vi "Pomiar_glowny.vi"() -> ()   [LabVIEW 2012]
panel:
  in  "stop":bool
  in  "Temp1":path
  in  "Temp2":path=path "D:/temperature2.txt"
  out "Temp 2 °C]":dbl format="%#_4g"
  out "Temp2 Chart":dbl(graph) caption="Temperature Chart"
  out "error out 2":errorcluster
  out "error out":errorcluster
  out "id":bool
  out "crc":bool
  out "Voltage [V]":dbl format="%#_2g"
  out "Potentiometer":dbl(knob) scale=0.0..3.0
  out "Temp1 Chart":dbl(graph) caption="Temperature Chart"
  out "Temp1 °C]":dbl format="%#_4g"
  out "Temp1":dbl(slide) scale=-40.0..120.0
  in  "Serial Port":refnum<visa-resource-name>="COM6"
  in  "stop":bool
  out "Received":string
  in  "?":bool
  # "POMIAR WARTOŒCI ANALOGOWYCH"
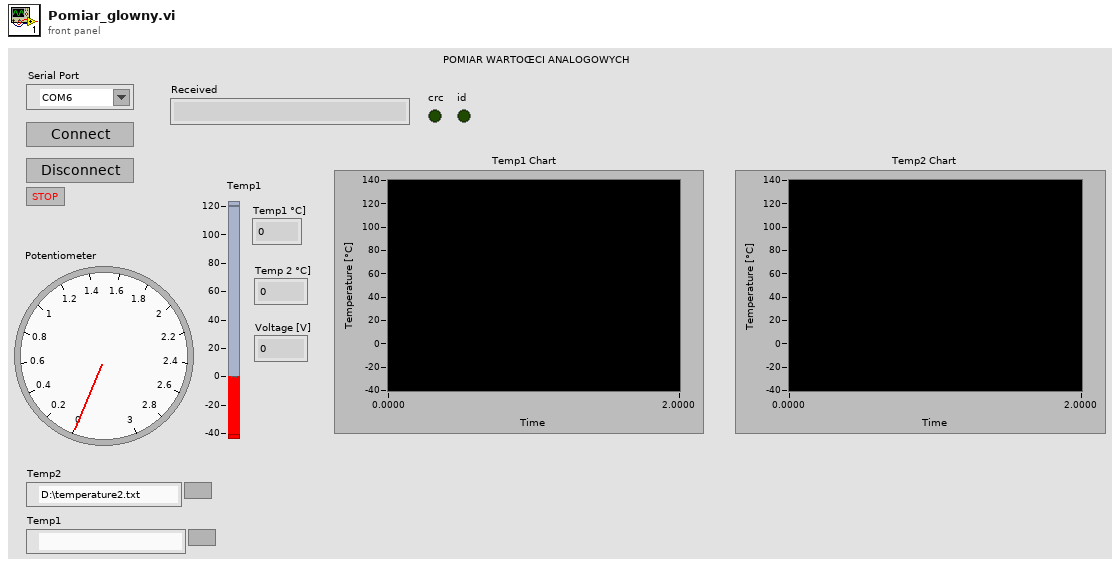
[diagram p1: front panel]
types:
  T1 = enum16{"open", "replace", "create", "open or create", "replace or create", "replace or create with confirmation"}
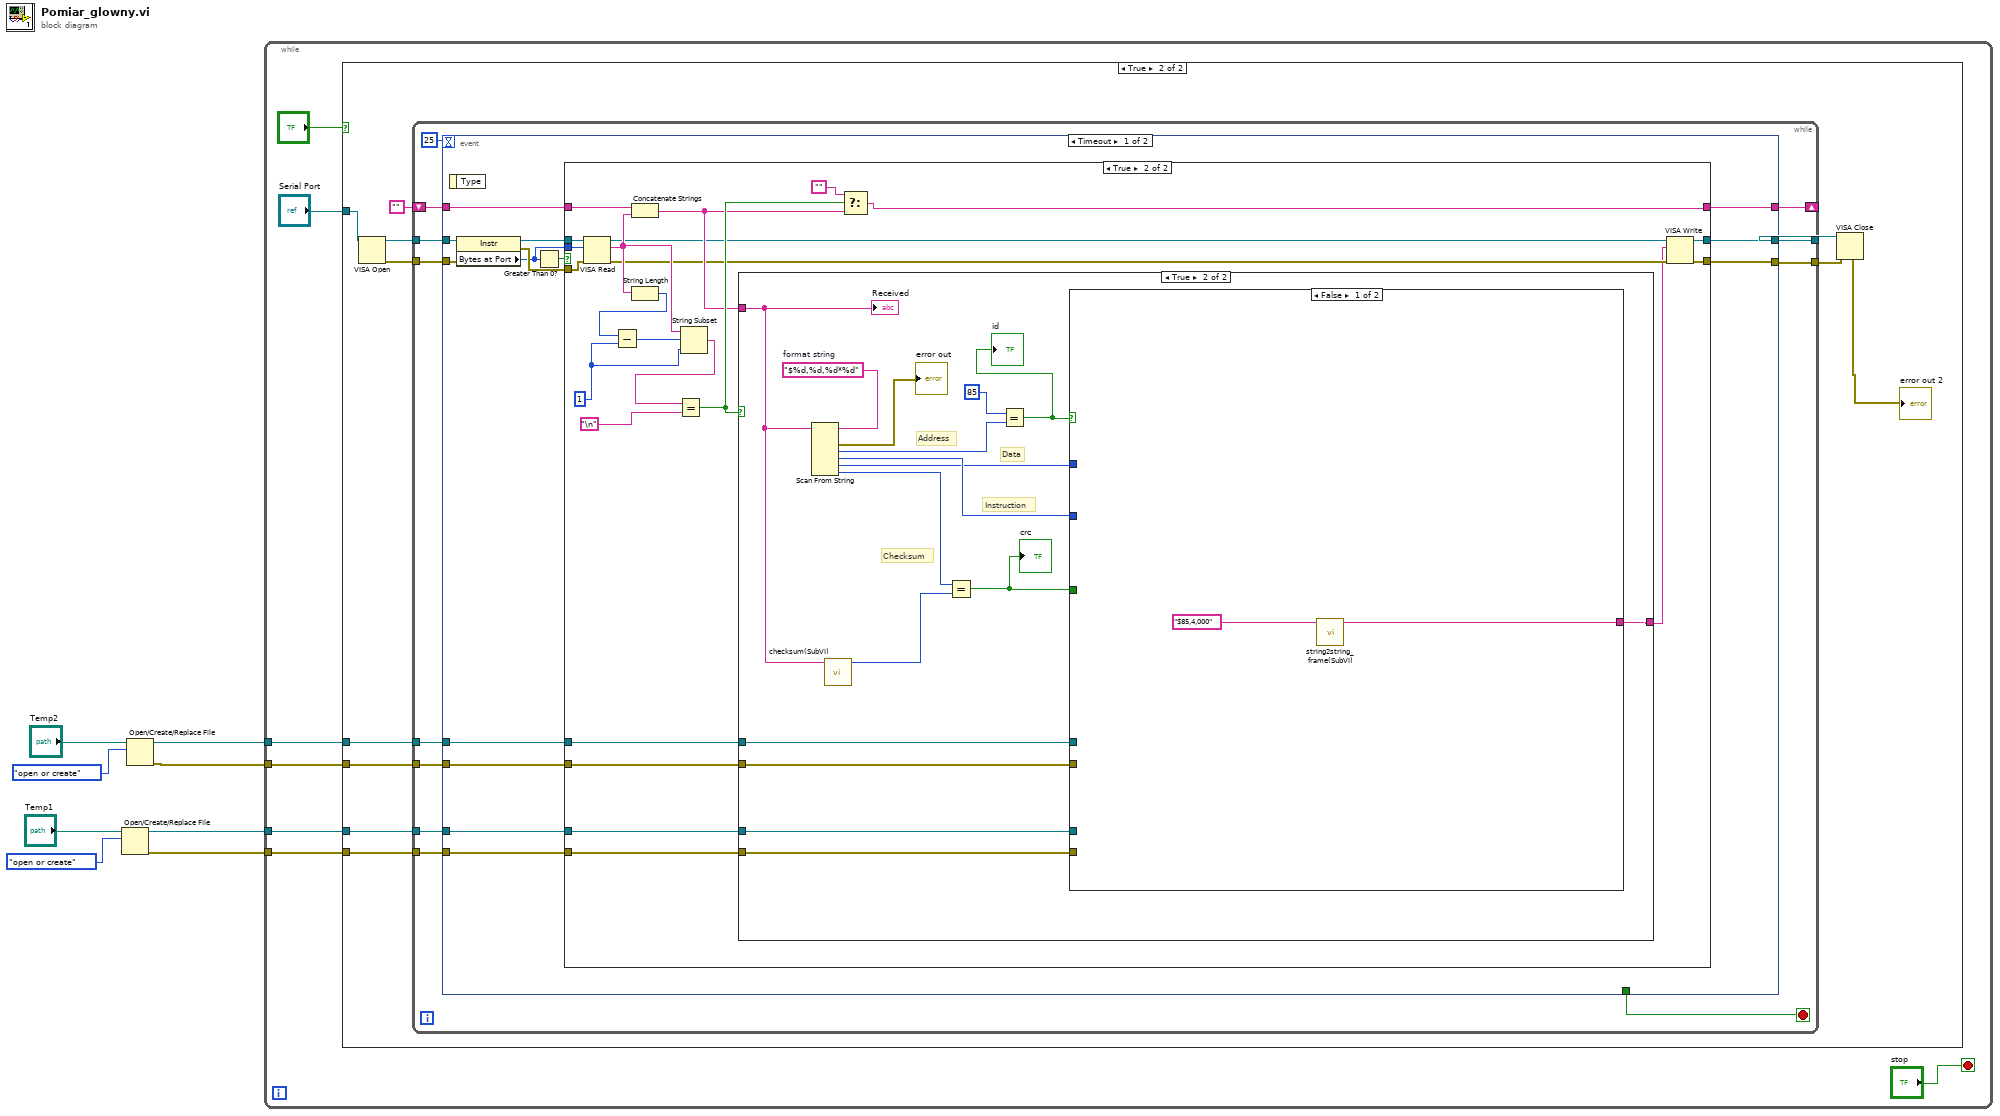
[diagram p0: block diagram]
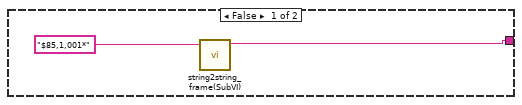
[diagram p4: hidden frame]
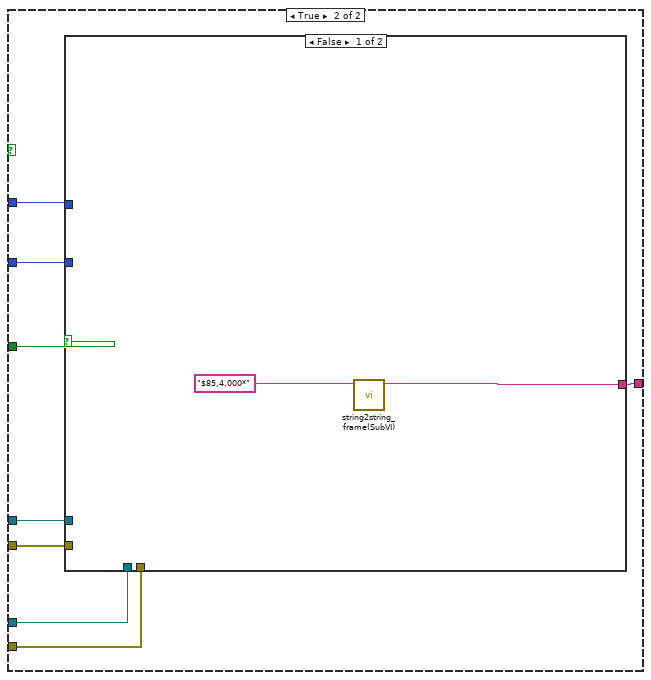
[diagram p5: hidden frame]
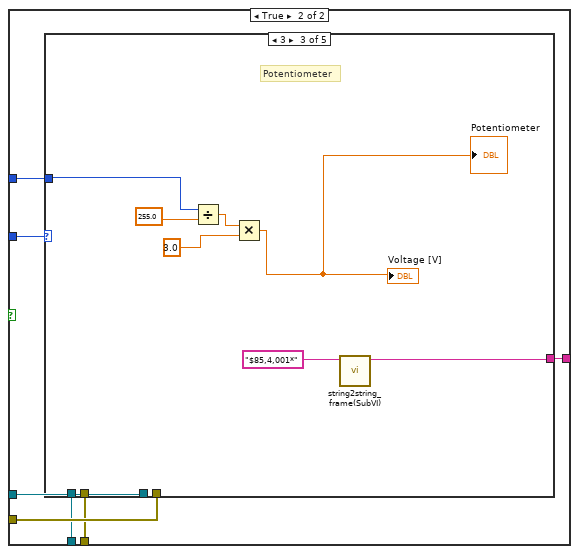
[diagram p6: hidden frame]
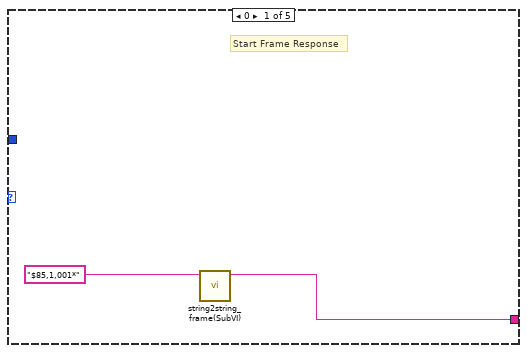
[diagram p7: hidden frame]
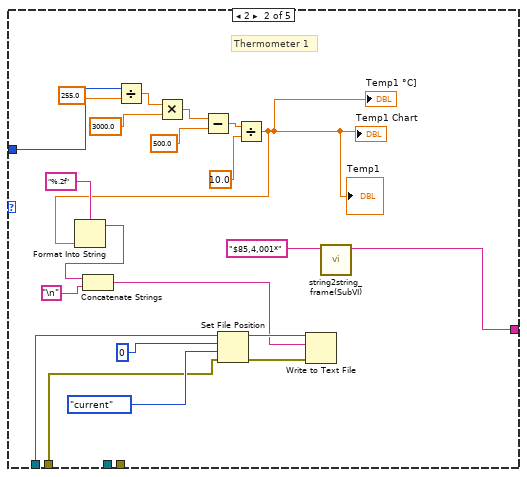
[diagram p8: hidden frame]
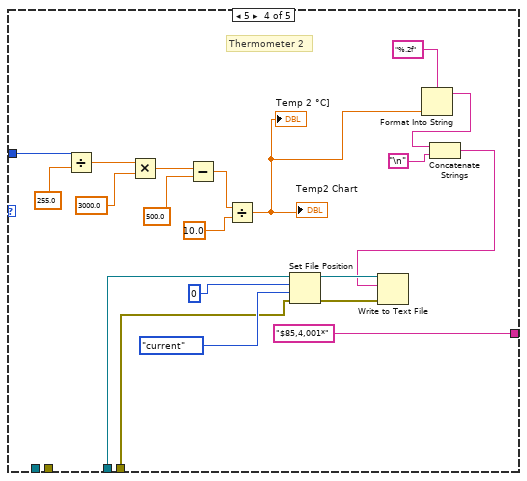
[diagram p9: hidden frame]
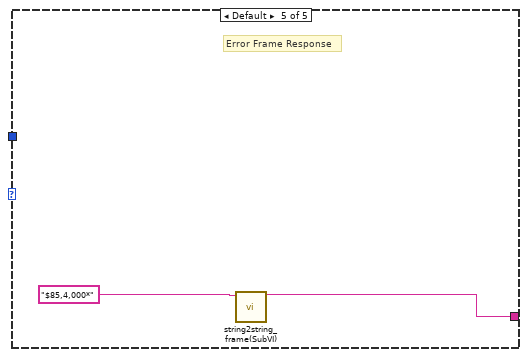
[diagram p10: hidden frame]
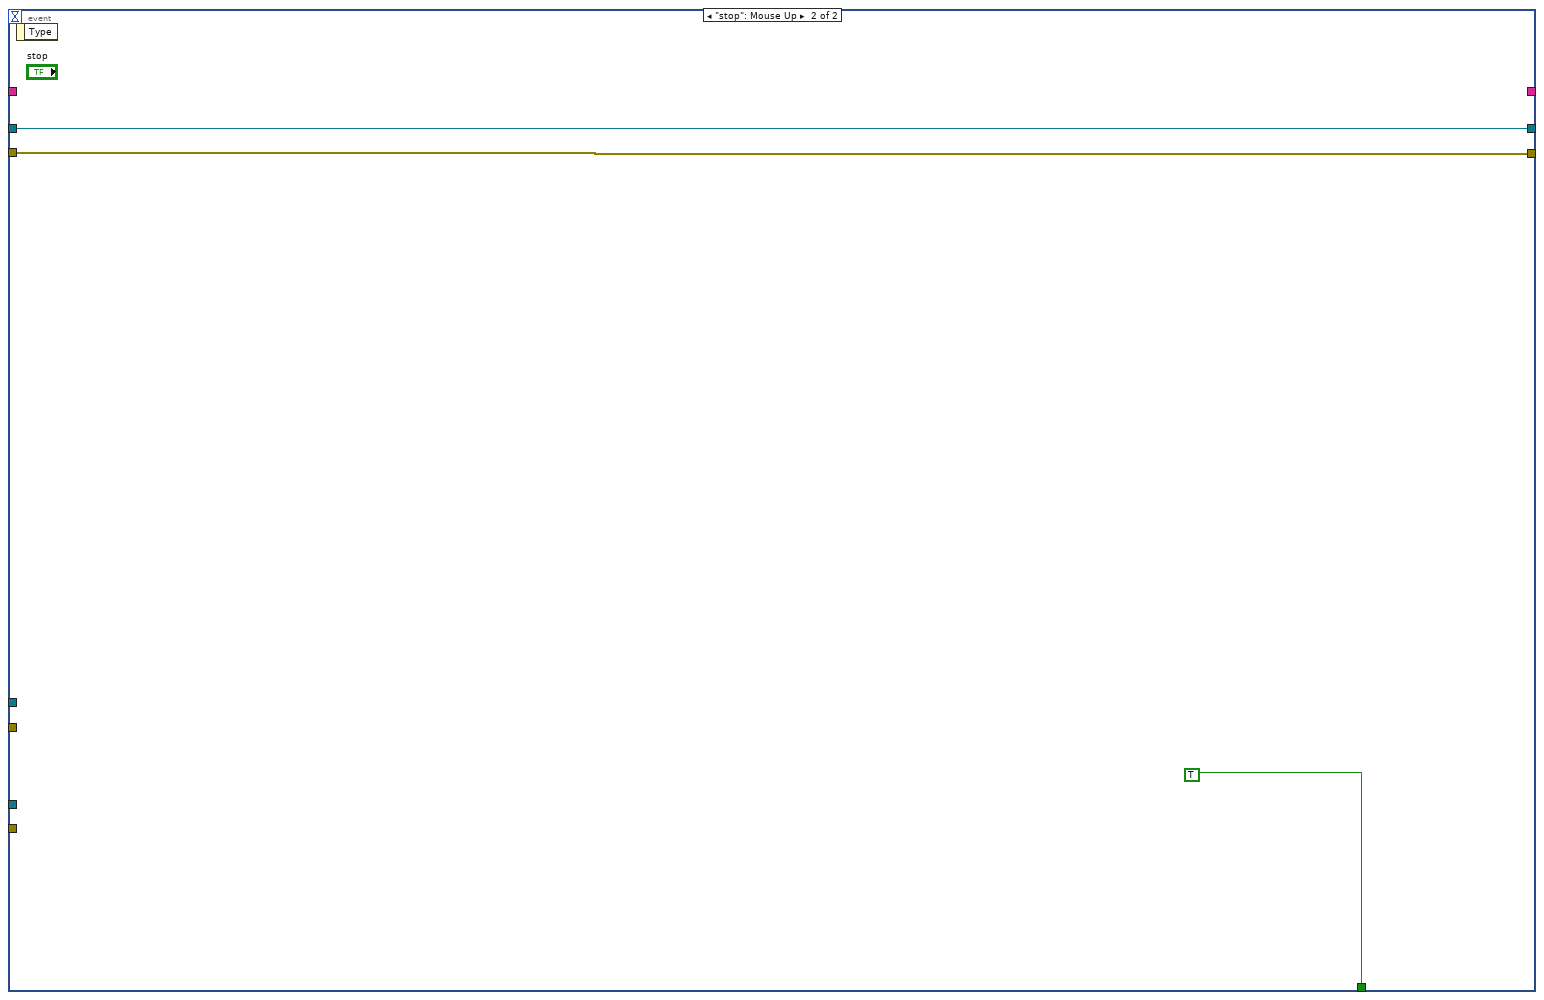
[diagram p11: hidden frame]
diagram:
  n1 = Open/Create/Replace File(file path (use dialog)="Temp1", operation (0:open)=T1."open or create") -> (refnum out=w2:refnum<file>, error out=w1:errorcluster)  [unwired: 4 in, 1 out]
  n2 = Open/Create/Replace File(file path (use dialog)="Temp2", operation (0:open)=T1."open or create") -> (refnum out=w6:refnum<file>, error out=w5:errorcluster)  [unwired: 4 in, 1 out]
  n3 = while {
    tunnel: w6 -> [w13]
    tunnel: w5 -> [w12]
    tunnel: w2 -> [w11]
    tunnel: w1 -> [w10]
    stop <- "stop" stop-if-true
    n4 = case shown="True" "?" {
      tunnel: "Serial Port" -> [_ w21]
      tunnel: w13 -> [_ w19]
      tunnel: w12 -> [_ w18]
      tunnel: w11 -> [_ w17]
      tunnel: w10 -> [_ w16]
      frame False {
      }
      frame True {
        n5 = VISA Open(VISA resource name=w21) -> (VISA resource name=w24:refnum<visa-resource-name>, error out=w23:errorcluster)  [unwired: 4 in]
        n6 = while {
          tunnel: w24 -> [w38]
          tunnel: [w37] -> w26
          tunnel: w23 -> [w35]
          tunnel: [w34] -> w25
          shift-right: [w32] -> _
          shift-left: "" -> [w33]
          tunnel: w19 -> [w30]
          tunnel: w18 -> [w29]
          tunnel: w17 -> [w28]
          tunnel: w16 -> [w27]
          stop <- w31 stop-if-true
          n7 = event shown="[0] Timeout" {
            selector: _ -> [_ _]
            dyn-events: _ -> [_ _]
            timeout: 25 ("millisecond multiple") -> [_ _]
            tunnel: w38 -> [w51 w170]
            tunnel: [w44 w170] -> w37
            tunnel: [_ TRUE] -> w31
            tunnel: w35 -> [w47 w168]
            tunnel: [w43 w168] -> w34
            tunnel: w33 -> [w46 _]
            tunnel: [w45 _] -> w32
            tunnel: w30 -> [w42 _]
            tunnel: w29 -> [w41 _]
            tunnel: w28 -> [w40 _]
            tunnel: w27 -> [w39 _]
            event Timeout {
              n8 = event-data() -> ()  [unwired: 1 in, 1 out]
              n9 = property class="Instr"(reference=w51, error in=w47) -> (reference out=w50:refnum<visa-resource-name>, error out=w52:errorcluster, "Bytes at Port"=w48:u32)
              n10 = Greater Than 0?(x=w48) -> (x > 0?=w49:bool)
              n11 = case shown="True" w49 {
                tunnel: w50 -> [w55 w78]
                tunnel: w48 -> [_ w77]
                tunnel: [w55 w64] -> w44
                tunnel: w52 -> [w53 w73]
                tunnel: w46 -> [w54 w72]
                tunnel: [w54 w70] -> w45
                tunnel: [w53 w63] -> w43
                tunnel: w42 -> [_ w59]
                tunnel: w41 -> [_ w58]
                tunnel: w40 -> [_ w57]
                tunnel: w39 -> [_ w56]
                frame False {
                }
                frame True {
                  w75 = 1 ("length (rest)")
                  n12 = VISA Read(VISA resource name=w78, byte count=w77, error in (no error)=w73) -> (VISA resource name out=w62:refnum<visa-resource-name>, read buffer=w74:string, error out=w61:errorcluster)  [unwired: 1 out]
                  n13 = Concatenate Strings(w72, w74) -> (w68:string)
                  n14 = String Length(string=w74) -> (length=w67:i32)
                  n15 = Subtract(x=w67, y=w75) -> (x-y=w76:i32)
                  n16 = String Subset(string=w74, offset (0)=w76, length (rest)=w75) -> (substring=w66:string)
                  n17 = Equal?(x=w66, y="\n") -> (x = y?=w69:bool)
                  n18 = case shown="True" w69 {
                    tunnel: w68 -> [_ w92]
                    tunnel: [w79 w88] -> w60
                    tunnel: w59 -> [_ w84]
                    tunnel: w58 -> [_ w83]
                    tunnel: w57 -> [_ w82]
                    tunnel: w56 -> [_ w81]
                    frame False {
                      n19 = call "string2string_frame(SubVI).vi"("String in"="$85,1,001*") -> ("String out"=w79:string)  [unwired: 10 in]
                    }
                    frame True {
                      w96 = "$%d,%d,%d*%d"  # format string
                      # "Checksum"
                      # "Instruction"
                      # "Data"
                      # "Address"
                      n20 = Scan From String(format string=w96, input string=w92) -> (error out=→"error out":errorcluster, output 1=w94:i32, output 2=w93:i32, output 3=w87:i32, output 4=w91:i32)  [unwired: 6 in, 2 out]
                      n21 = call "checksum(SubVI).vi"("String"=w92) -> ("Numeric"=w89:u8)  [unwired: 10 in]
                      n22 = Equal?(x=w91, y=w89) -> (x = y?=w86:bool)
                      "crc" <- w86
                      n23 = Equal?(x=85, y=w94) -> (x = y?=w90:bool)
                      "id" <- w90
                      n24 = case shown="False" w90 {
                        tunnel: w93 -> [_ w105]
                        tunnel: w87 -> [_ w106]
                        tunnel: w86 -> [_ w103]
                        tunnel: [w97 w104] -> w88
                        tunnel: w84 -> [_ w102]
                        tunnel: w83 -> [_ w101]
                        tunnel: w82 -> [_ w100]
                        tunnel: w81 -> [_ w99]
                        frame False {
                          n25 = call "string2string_frame(SubVI).vi"("String in"="$85,4,000") -> ("String out"=w97:string)  [unwired: 10 in]
                        }
                        frame True {
                          n26 = case shown="False" w103 {
                            tunnel: w106 -> [_ w115]
                            tunnel: w105 -> [_ w114]
                            tunnel: [w107 w113] -> w104
                            tunnel: w102 -> [_ w112]
                            tunnel: w101 -> [_ w111]
                            tunnel: w100 -> [_ w110]
                            tunnel: w99 -> [_ w109]
                            frame False {
                              n27 = call "string2string_frame(SubVI).vi"("String in"="$85,4,000*") -> ("String out"=w107:string)  [unwired: 10 in]
                            }
                            frame True {
                              n28 = case shown="3" w114 {
                                tunnel: w115 -> [_ w129 w140 w158 _]
                                tunnel: [w116 w131 w141 "$85,4,001*" w167] -> w113
                                tunnel: w112 -> [_ _ _ w148 _]
                                tunnel: w111 -> [_ _ _ w147 _]
                                tunnel: w110 -> [_ w124 _ _ _]
                                tunnel: w109 -> [_ w123 _ _ _]
                                frame 0 {
                                # "Start Frame Response"
                                n29 = call "string2string_frame(SubVI).vi"("String in"="$85,1,001*") -> ("String out"=w116:string)  [unwired: 10 in]
                                }
                                frame 2 {
                                # "Thermometer 1"
                                n30 = Divide(x=w129, y=255.0) -> (x/y=w137:dbl)
                                n31 = Multiply(x=w137, y=3000.0) -> (x*y=w135:dbl)
                                n32 = Subtract(x=w135, y=500.0) -> (x-y=w132:dbl)
                                n33 = Set File Position(offset (in bytes) (0)=u32 0 ("millisecond multiple"), refnum=w124, from (0:start)=enum16{"start", "end", "current"}."current", error in=w123) -> (refnum out=w126:refnum<file>, error out=w125:errorcluster)
                                n34 = Divide(x=w132, y=10.0) -> (x/y=w119:dbl)
                                "Temp1 Chart" <- w119
                                "Temp1 °C]" <- w119
                                "Temp1" <- w119
                                n35 = Format Into String(format string="%.2f", w119) -> (resulting string=w121:string)  [unwired: 2 in, 1 out]
                                n36 = Concatenate Strings(w121, "\n" ("Line Feed Constant")) -> (w118:string)
                                n37 = Write to Text File(file (use dialog)=w126, text=w118, error in=w125) -> ()  [unwired: 1 in, 3 out]
                                n38 = call "string2string_frame(SubVI).vi"("String in"="$85,4,001*") -> ("String out"=w131:string)  [unwired: 10 in]
                                }
                                frame 3 {
                                # "Potentiometer"
                                n39 = Divide(x=w140, y=255.0) -> (x/y=w144:dbl)
                                n40 = Multiply(x=w144, y=3.0) -> (x*y=→"Voltage [V]" →"Potentiometer":dbl)
                                n41 = call "string2string_frame(SubVI).vi"("String in"="$85,4,001*") -> ("String out"=w141:string)  [unwired: 10 in]
                                }
                                frame 5 {
                                # "Thermometer 2"
                                n42 = Divide(x=w158, y=255.0) -> (x/y=w164:dbl)
                                n43 = Multiply(x=w164, y=3000.0) -> (x*y=w162:dbl)
                                n44 = Subtract(x=w162, y=500.0) -> (x-y=w159:dbl)
                                n45 = Divide(x=w159, y=10.0) -> (x/y=w146:dbl)
                                "Temp2 Chart" <- w146
                                "Temp 2 °C]" <- w146
                                n46 = Set File Position(offset (in bytes) (0)=u32 0 ("millisecond multiple"), refnum=w148, from (0:start)=enum16{"start", "end", "current"}."current", error in=w147) -> (refnum out=w154:refnum<file>, error out=w153:errorcluster)
                                n47 = Format Into String(format string="%.2f", w146) -> (resulting string=w151:string)  [unwired: 2 in, 1 out]
                                n48 = Concatenate Strings(w151, "\n" ("Line Feed Constant")) -> (w149:string)
                                n49 = Write to Text File(file (use dialog)=w154, text=w149, error in=w153) -> ()  [unwired: 1 in, 3 out]
                                }
                                frame Default {
                                # "Error Frame Response"
                                n50 = call "string2string_frame(SubVI).vi"("String in"="$85,4,000*") -> ("String out"=w167:string)  [unwired: 10 in]
                                }
                              }
                            }
                          }
                        }
                      }
                      "Received" <- w92
                    }
                  }
                  n51 = Select(t="", s=w69, f=w68) -> (s? t:f=w70:string)
                  n52 = VISA Write(VISA resource name=w62, write buffer=w60, error in (no error)=w61) -> (VISA resource name out=w64:refnum<visa-resource-name>, error out=w63:errorcluster)  [unwired: 1 out]
                }
              }
            }
            event "stop": Mouse Up {
              n53 = event-data() -> ()  [unwired: 1 in, 1 out]
            }
          }
        }
        n54 = VISA Close(VISA resource name=w26, error in (no error)=w25) -> (error out=→"error out 2":errorcluster)
      }
    }
  }
